vi "Get Twiddle Factors from BRAM (U16 Address) SGL Output.vi"(7 "FFT Size":T1=enum."8192", 8 "Input Data Valid":bool, 9 "Reset?":bool) -> (0 "Output Valid":bool, 1 "phase_out":fxp<+/-,16,1> format="%.14g", 2 "Output":T2)   [LabVIEW 2011]
doc: "This VI generates twiddle factors for sine and cosine generation\n\n<b> Latency = 19 Ticks </b>"
uses:
  <userlib>/FPGA Library/Code Development/Signal Processing/FFT Block/FFT/FFT Size.ctl
  <vilib>/rvi/FXPMathLib/FxpConvert/subVIs/nifxpmath_Convert_SimConfig.ctl
  <vilib>/fxp/LVFixedPointQuantizationPolicyTypeDef.ctl
  <vilib>/fxp/LVFixedPointOverflowPolicyTypeDef.ctl
  <vilib>/rvi/FXPMathLib/FxpConvert/simVIs/DllFxpConvertTemp_sub.vi
  <vilib>/rvi/IPIntegrationNode/IPINode_Utilities/niFpgaIPINodeSimCore.vi
  <vilib>/rvi/FXPMathLib/basic elements/FxpDiscreteDelay/XNode/nifxpmath_DiscreteDelay.xnode
  <vilib>/rvi/FXPMathLib/FxpInterpret/XNode/nifxpmath_Interpret.xnode
  <vilib>/rvi/FXPMathLib/FxpConvert/XNode/nifxpmath_Convert.xnode
  <vilib>/rvi/XilinxIP/XIPIN_XNode/niFpgaXIPIN.xnode
  <userlib>/FPGA Library/Code Development/Signal Processing/FFT Block/Twiddle Factor/LUT/SinCosLUT_4AF2FDD64E94328E5B0A30B3AC6E6500.dll
  <vilib>/rvi/IPIntegrationNode/IPINode_Xnode/niFpgaIPINode.xnode
  <userlib>/FPGA Library/Code Development/Signal Processing/FFT Block/Twiddle Factor/FXPtoFLoat/fxptosgl_3543ACB549D8B4526FD3C69EA9E8368A.dll
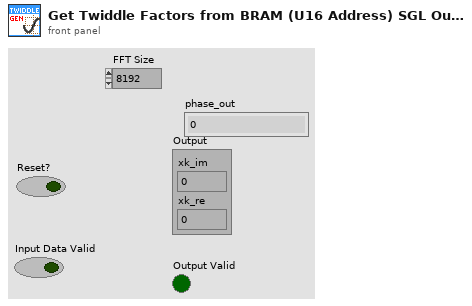
[diagram p1: front panel]
types:
  T1 = typedef "FFT Size.ctl" = enum16{"32", "64", "128", "256", "512", "1024", "2048", "4096", "8192", "16384", "32768", "65536"}
  T2 = cluster{"xk_im":fxp<+,32,32>, "xk_re":fxp<+,32,32>}
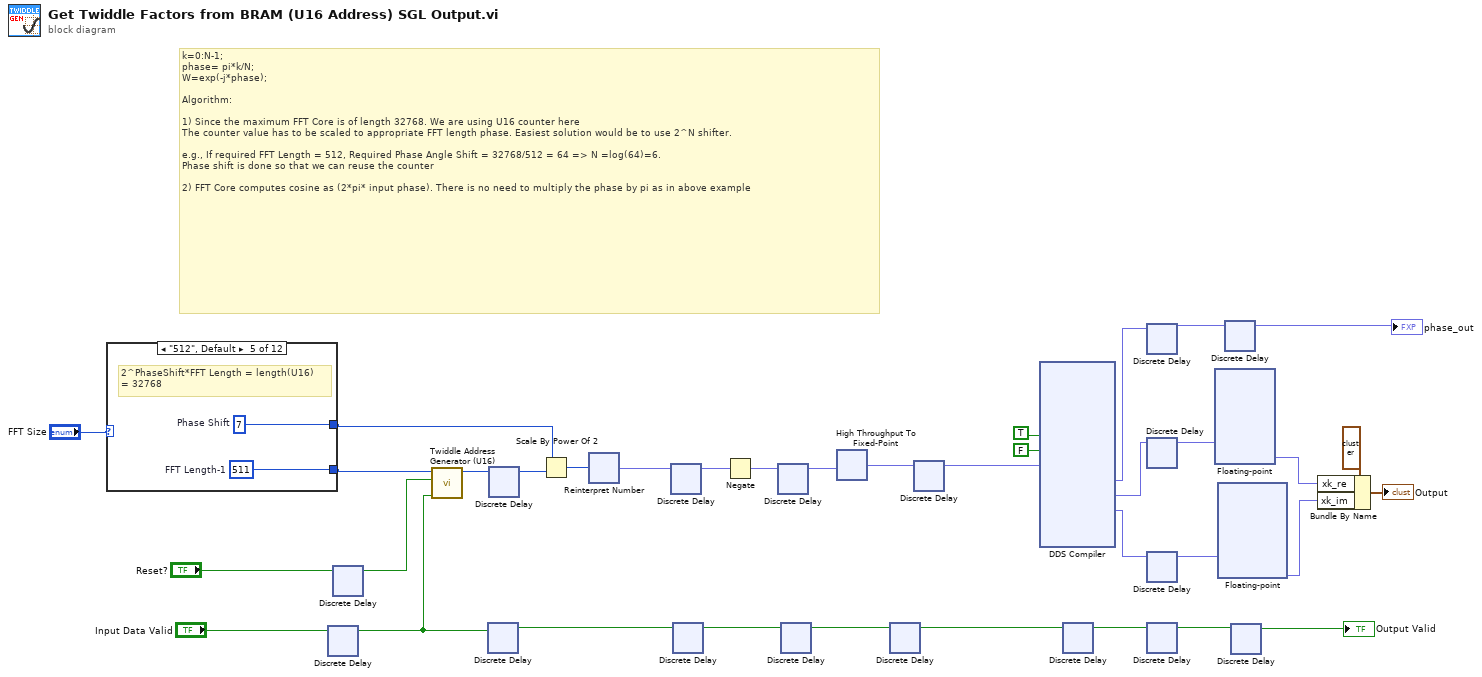
[diagram p0: block diagram]
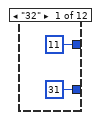
[diagram p2: hidden frame]
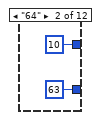
[diagram p3: hidden frame]
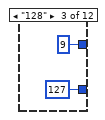
[diagram p4: hidden frame]
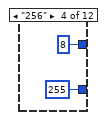
[diagram p5: hidden frame]
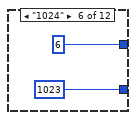
[diagram p6: hidden frame]
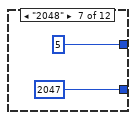
[diagram p7: hidden frame]
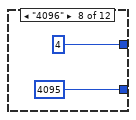
[diagram p8: hidden frame]
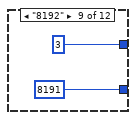
[diagram p9: hidden frame]
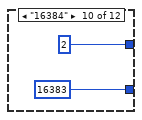
[diagram p10: hidden frame]
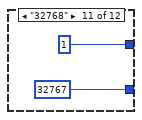
[diagram p11: hidden frame]
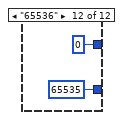
[diagram p12: hidden frame]
diagram:
  # "k=0:N-1;\nphase= pi*k/N;\nW=exp(-j*phase);\n\nAlgorithm:\n\n1) Since the maximum FFT Core is of length 32768. We are using U16 counter here\nThe counter value has to be scaled to appropriate FFT length phase. Easiest solution would be to use 2^N shifter.\n\ne.g., If required FFT Length = 512, Required Phase Angle Shift = 32768/512 = 64 => N =log(64)=6.\nPhase shift is done so that we can reuse the counter\n\n2) FFT Core computes cosine as (2*pi* input phase). There is no need to multiply the phase by pi as in above example"
  n1 = case shown="\"512\", Default" "FFT Size" {
    tunnel: [u8 11 ("n") u8 10 ("n") u8 9 ("n") u8 8 ("n") w46 u8 6 ("n") u8 5 ("n") u8 4 ("n") u8 3 ("n") u8 2 ("n") u8 1 ("n") u8 0 ("n")] -> w2
    tunnel: [u16 31 ("FFT Length-1") u16 63 ("FFT Length-1") u16 127 ("FFT Length-1") u16 255 ("FFT Length-1") w45 u16 1023 u16 2047 u16 4095 u16 8191 u16 16383 u16 32767 u16 65535 ("FFT Length-1")] -> w1
    frame "32" {
    }
    frame "64" {
    }
    frame "128" {
    }
    frame "256" {
    }
    frame "512", Default {
      w45 = u16 511  # FFT Length-1
      w46 = u8 7  # Phase Shift
      # "2^PhaseShift*FFT Length = length(U16)\n= 32768"
    }
    frame "1024" {
    }
    frame "2048" {
    }
    frame "4096" {
    }
    frame "8192" {
    }
    frame "16384" {
    }
    frame "32768" {
    }
    frame "65536" {
    }
  }
  n2 = xnode "Discrete Delay"("D"="Input Data Valid") -> ("Q"=w28:bool)
  n3 = xnode "Discrete Delay"("D"="Reset?") -> ("Q"=w27:bool)
  n4 = call <userlib>:"Twiddle Address Generator (U16).vi"("INC?"=w28, "Reset?"=w27, "rollover"=w1) -> ("count"=w35:u16)  [unwired: 8 in]
  n5 = xnode "Discrete Delay"("D"=w28) -> ("Q"=w25:bool)
  n6 = xnode "Discrete Delay"("D"=w35) -> ("Q"=w26:u16)
  n7 = Scale By Power Of 2(n=w2, x=w26) -> (x*2^n=w33:u16)
  n8 = xnode "Reinterpret Number"("x"=w33) -> ("y"=w15:fxp<+,16,0>)
  n9 = xnode "Discrete Delay"("D"=w15) -> ("Q"=w30:fxp<+,16,0>)
  n10 = xnode "Discrete Delay"("D"=w25) -> ("Q"=w29:bool)
  n11 = Negate(x=w30) -> (-x=w13:fxp<+/-,17,1>)
  n12 = xnode "Discrete Delay"("D"=w13) -> ("Q"=w11:fxp<+/-,17,1>)
  n13 = xnode "Discrete Delay"("D"=w29) -> ("Q"=w10:bool)
  n14 = xnode "High Throughput To Fixed-Point"("x"=w11) -> ("y"=w12:fxp<+/-,16,1>)
  n15 = xnode "Discrete Delay"("D"=w10) -> ("Q"=w8:bool)
  n16 = xnode "Discrete Delay"("D"=w12) -> ("Q"=w9:fxp<+/-,16,1>)
  n17 = xnode ("DDS Compiler")("ce"=TRUE, "sclr"=FALSE, "phase_in"=w9) -> ("phase_out"=w16:fxp<+/-,16,1>, "cosine"=w19:fxp<+/-,18,2>, "sine"=w14:fxp<+/-,18,2>)  [unwired: 2 out]
  n18 = xnode "Discrete Delay"("D"=w8) -> ("Q"=w18:bool)
  n19 = xnode "Discrete Delay"("D"=w16) -> ("Q"=w6:fxp<+/-,16,1>)
  n20 = xnode "Discrete Delay"("D"=w19) -> ("Q"=w7:fxp<+/-,18,2>)
  n21 = xnode "Discrete Delay"("D"=w14) -> ("Q"=w5:fxp<+/-,18,2>)
  n22 = xnode "Discrete Delay"("D"=w18) -> ("Q"=w4:bool)
  n23 = xnode ("Floating-point")("a"=w7) -> ("result"=w23:fxp<+,32,32>)
  n24 = xnode ("Floating-point")("a"=w5) -> ("result"=w22:fxp<+,32,32>)
  n25 = xnode "Discrete Delay"("D"=w6) -> ("Q"=→"phase_out":fxp<+/-,16,1>)
  n26 = xnode "Discrete Delay"("D"=w4) -> ("Q"=→"Output Valid":bool)
  n27 = Bundle By Name(cluster=T2 {"xk_im"=0.0, "xk_re"=0.0} ("FFT Output"), "xk_re"=w23, "xk_im"=w22) -> (→"Output":T2)
